vi "Generator_b.vi"(0 "Stop":bool caption="Start/Stop") -> (4 "Generated_Data":dbl caption="Generated Data")   [LabVIEW 2023]
doc: "This VI continuously generate Data and push it to the Acquisition VI.\nTransfer of thet data happens under Simple LV2."
uses:
  Controls/Operation_Simple_LV2.ctl
  <vilib>/numeric/Random Number (Range) DBL.vi
panel:
  out "Error_Out":errorcluster
  in  "Error_In":errorcluster
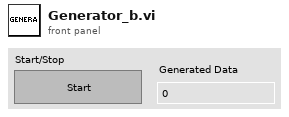
[diagram p1: front panel]
types:
  T1 = typedef "Operation_Simple_LV2.ctl" = enum16{"Write", "Read"}
  T2 = enum16{"Left Button", "Center Button", "Right Button", "Window Close"}
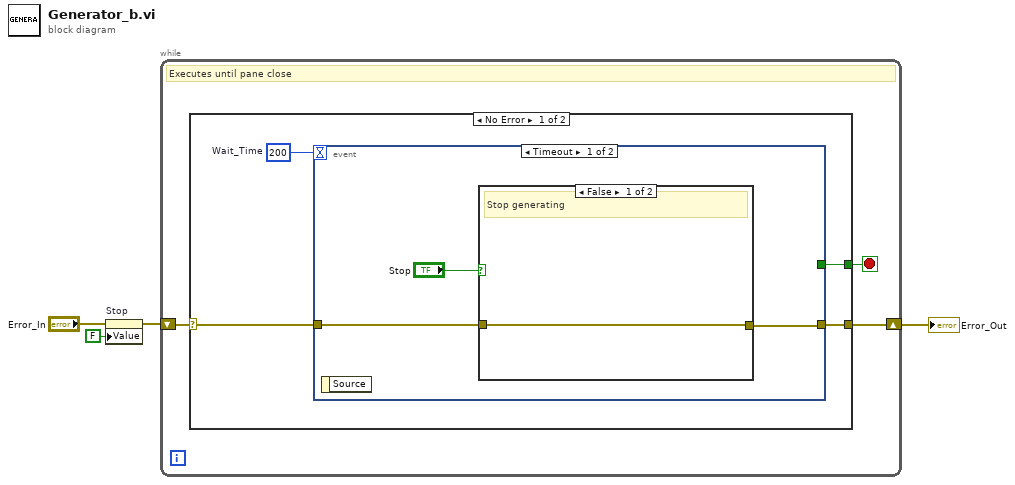
[diagram p0: block diagram]
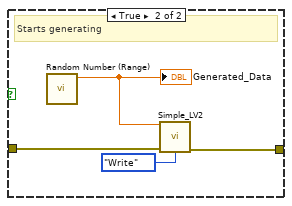
[diagram p2: hidden frame]
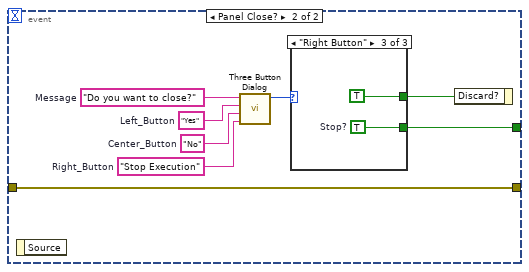
[diagram p3: hidden frame]
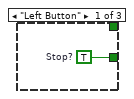
[diagram p4: hidden frame]
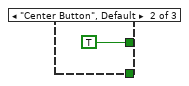
[diagram p5: hidden frame]
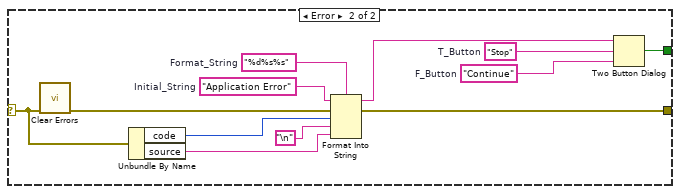
[diagram p6: hidden frame]
diagram:
  n1 = property on="Stop" class="Bool (strict)"(error in="Error_In", "Value"=FALSE ("Stop")) -> (error out=w3:errorcluster)  [unwired: 1 in, 1 out]
  n2 = while {
    shift-right: [w5] -> w4
    shift-left: w3 -> [w6]
    stop <- w7 stop-if-true
    # "Executes until pane close"
    n3 = case shown="No Error" w6 {
      selector: w6 -> [w9 w33]
      tunnel: [w10 w32] -> w7
      tunnel: [w8 w34] -> w5
      frame No Error {
        w11 = 200  # Wait_Time
        n4 = event shown="[0] Timeout" {
          selector: _ -> [_ _]
          dyn-events: _ -> [_ _]
          timeout: w11 -> [_ _]
          tunnel: [_ w21] -> w10
          tunnel: w9 -> [w14 w20]
          tunnel: [w13 w20] -> w8
          event Timeout {
            n5 = event-data() -> ()  [unwired: 1 in, 1 out]
            n6 = case shown="False" "Stop" {
              tunnel: w14 -> [w15 w18]
              tunnel: [w15 w17] -> w13
              frame False {
                # "Stop generating"
              }
              frame True {
                # "Starts generating"
                n7 = call-poly <vilib>:"Random Number (Range).vi"() -> ("number"=w19:dbl)  [unwired: 11 in]
                "Generated_Data" <- w19
                n8 = call "Simple_LV2.vi"("Data_In"=w19, "Error_In"=w18, "Operation"=Operation_Simple_LV2."Write") -> ("Error_Out"=w17:errorcluster)  [unwired: 11 in, 1 out]
              }
            }
          }
          event Panel Close? {
            w24 = "Stop Execution"  # Right_Button
            w25 = "No"  # Center_Button
            w26 = "Yes"  # Left_Button
            w27 = "Do you want to close?"  # Message
            n9 = event-data() -> ()  [unwired: 1 in, 1 out]
            n10 = call <vilib>:"Three Button Dialog.vi"("Right Button Text (\"Cancel\")"=w24, "Center Button Text (\"No\")"=w25, "Left Button Text (\"Yes\")"=w26, "message"=w27) -> ("Which Button?"=w23:T2)  [unwired: 7 in]
            n11 = case shown="\"Right Button\"" w23 {
              tunnel: [_ TRUE ("Discard?") TRUE ("Discard?")] -> w22
              tunnel: [w28 _ w31] -> w21
              frame "Left Button" {
                w28 = TRUE  # Stop?
              }
              frame "Center Button", Default {
              }
              frame "Right Button" {
                w31 = TRUE  # Stop?
              }
            }
            n12 = event-data("Discard?"=w22) -> ()  [unwired: 1 in, 1 out]
          }
        }
      }
      frame Error {
        w39 = "%d%s%s"  # Format_String
        w40 = "Application Error"  # Initial_String
        w41 = "Stop"  # T_Button
        w42 = "Continue"  # F_Button
        n13 = call <vilib>:"Clear Errors.vi"("error in (no error)"=w33) -> ("error out"=w37:errorcluster)  [unwired: 5 in, 1 out]
        n14 = Unbundle By Name(w33) -> ("code"=w36:i32, "source"=w35:string)
        n15 = Format Into String(format string=w39, initial string=w40, error in=w37, w36, "\n", w35) -> (resulting string=w43:string, error out=w34:errorcluster)
        n16 = Two Button Dialog(message=w43, 1:w42, 2:w41) -> (T button?=w32:bool)
      }
    }
  }
  "Error_Out" <- w4
